vi "Test Comm.vi"() -> ()   [LabVIEW 2021]
uses:
  ChannelCommon/typedef/FIFO Config.ctl
  ChannelCommon/ChannelCommon.lvlib
  CIFChannels/Typedef/Direction.ctl
  CIFChannels/CIFChannels.lvclass
  CIF_NIChn_DAQ_Base.lvclass
  ChannelCommon/typedef/TimeStamps.ctl
  ChannelCommon/typedef/Datatype Waveform.ctl
  ChannelCommon/typedef/New FIFO Instance Response.ctl
panel:
  out "status":string
  out "pass":bool
  out "error out":errorcluster
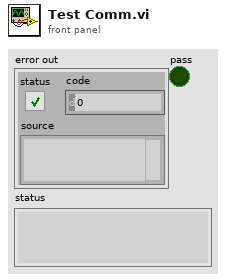
[diagram p1: front panel]
types:
  T1 = typedef "CIFChannels.lvclass/Direction.ctl" = enum16{"Publisher", "Subscriber"}
  T2 = typedef "ChannelCommon.lvlib/New FIFO Instance Response.ctl" = cluster{"Publisher":string, "Custom Data":u8[]}
  T3 = typedef "ChannelCommon.lvlib/TimeStamps.ctl" = cluster{"ClockID":u8, "T0":i64, "T_Out":i64}
  T4 = typedef "ChannelCommon.lvlib/FIFO Config.ctl" = cluster{"Max Bytes/Msg":u64, "Max Msg/FIFO":u64, "Flags":u64}
  T5 = typedef "ChannelCommon.lvlib/Datatype Waveform.ctl" = cluster{"Measurement":dbl[], "dT":dbl, "Timestamp":i64}
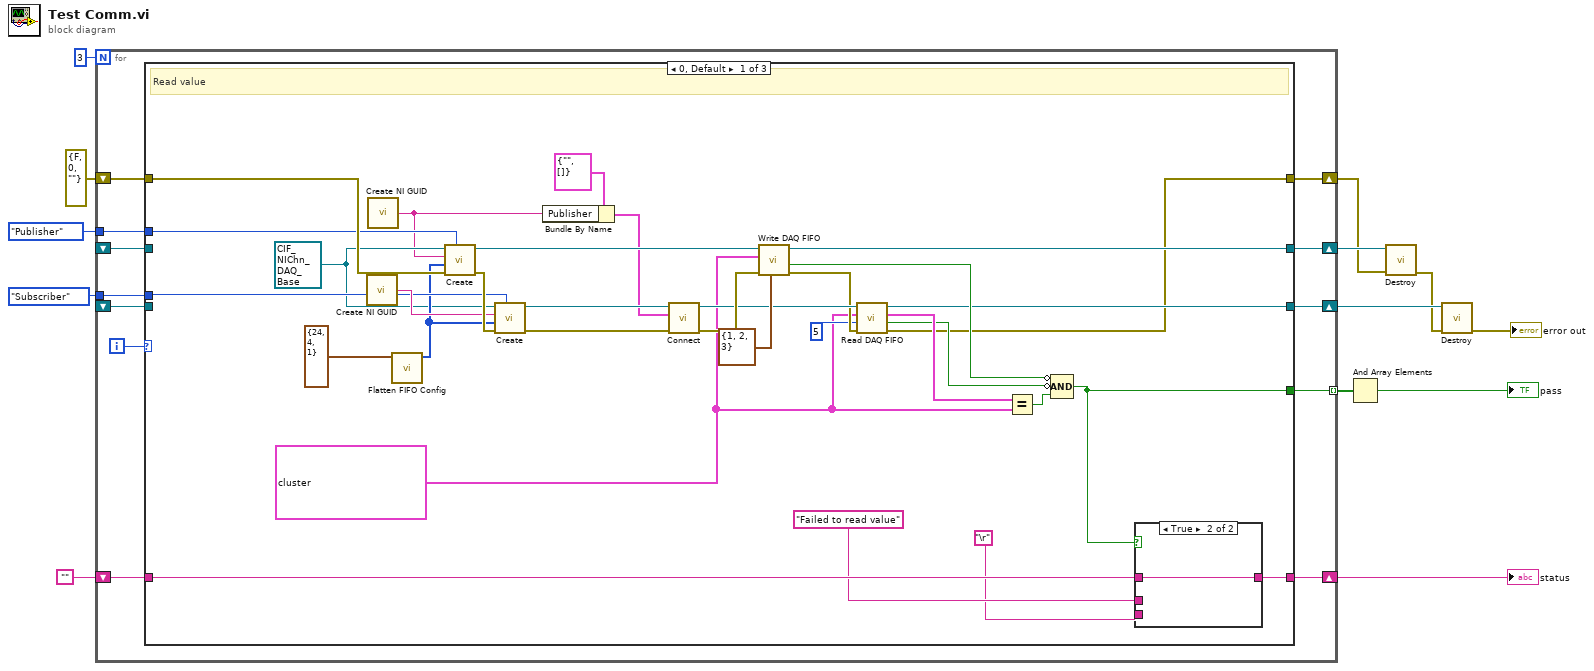
[diagram p0: block diagram]
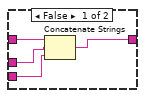
[diagram p2: hidden frame]
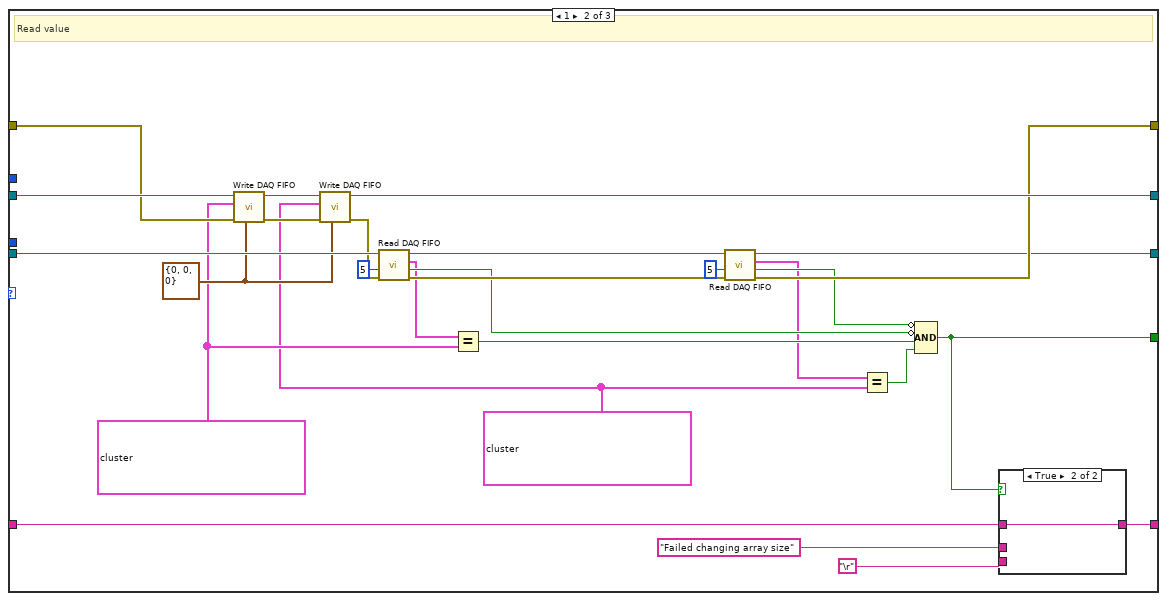
[diagram p3: hidden frame]
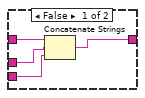
[diagram p4: hidden frame]
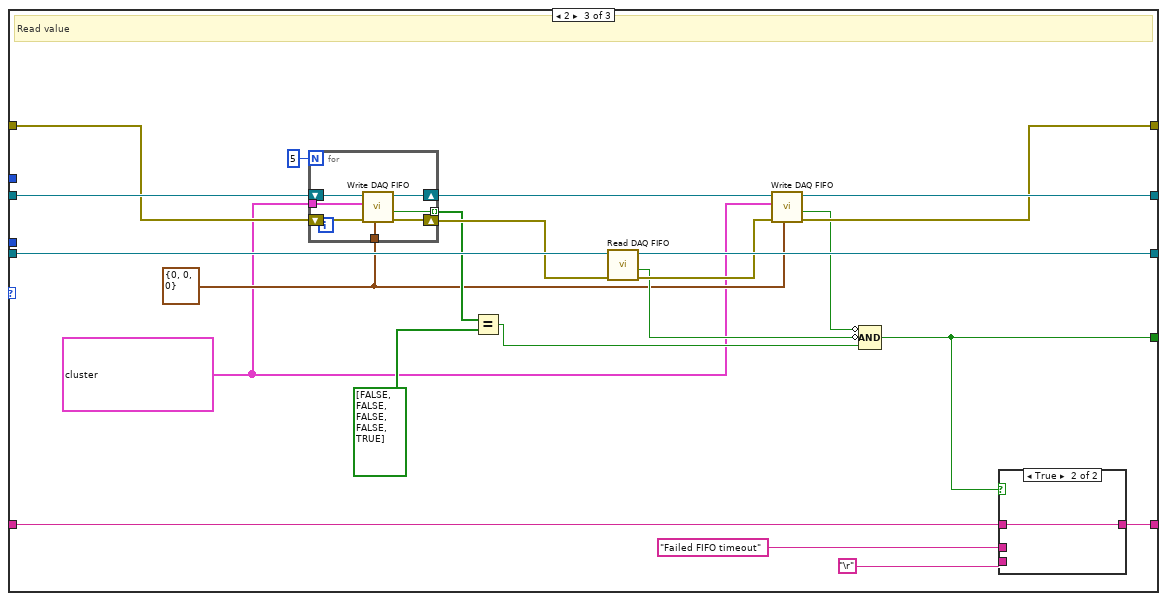
[diagram p5: hidden frame]
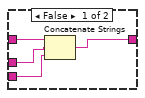
[diagram p6: hidden frame]
diagram:
  n1 = for {
    N: 3 -> [_]
    tunnel: [w25] -> w13 mode=indexing
    shift-right: [w14] -> w3
    shift-left: errorcluster {"status"=FALSE, "code"=0, "source"=""} ("error out") -> [w24]
    shift-right: [w21] -> w9
    shift-left: "" -> [w22]
    tunnel: Direction."Subscriber" ("Direction") -> [w20]
    tunnel: Direction."Publisher" ("Direction") -> [w19]
    shift-right: [w18] -> w5
    shift-left: _ -> [w16]
    shift-right: [w17] -> w4
    shift-left: _ -> [w15]
    i -> [w23]
    n2 = case shown="0, Default" w23 {
      tunnel: [w52 w85 w97] -> w25
      tunnel: w24 -> [w50 w81 w111]
      tunnel: [w30 w74 w103] -> w14
      tunnel: w22 -> [w57 w89 w116]
      tunnel: [w56 w88 w115] -> w21
      tunnel: w20 -> [w48 _ _]
      tunnel: w19 -> [w47 _ _]
      tunnel: [w32 w71 w108] -> w18
      tunnel: [w38 w78 w106] -> w17
      tunnel: w15 -> [_ w82 w112]
      tunnel: w16 -> [_ w77 w109]
      frame 0, Default {
        w42 = refnum<class "CIF_NIChn_DAQ_Base.lvclass"> refnum ("CIF_NIChn_FIFO_DAQ.lvclass")
        w29 = T5[] [{"Measurement"=array[986 elements], "dT"=43.0, "Timestamp"=2}, {"Measurement"=array[1001 elements], "dT"=34.0, "Timestamp"=1}] ("DAQ In")
        # "Read value"
        n3 = call <vilib>:"Create NI GUID.vi"() -> ("NI GUID"=w49:string)
        n4 = call <vilib>:"Create NI GUID.vi"() -> ("NI GUID"=w27:string)
        n5 = call "Flatten FIFO Config.vi"("FIFO Config in"=T4 {"Max Bytes/Msg"=24, "Max Msg/FIFO"=4, "Flags"=1}) -> ("Flattened FIFO Config"=w43:u8[])  [unwired: 10 in]
        n6 = call-dynamic "Create.vi"("Direction"=w47, "error in (no error)"=w50, "Custom Config Data"=w43, "Name"=w27, "CIF_NIChn_FIFO_DAQ in"=w42) -> ("error out"=w51:errorcluster, "CIF_NIChn_FIFO_DAQ out"=w41:refnum<class "CIF_NIChn_DAQ_Base.lvclass">)  [unwired: 5 in]
        n7 = call-dynamic "Create.vi"("Direction"=w48, "error in (no error)"=w51, "Custom Config Data"=w43, "Name"=w49, "CIF_NIChn_FIFO_DAQ in"=w42) -> ("error out"=w45:errorcluster, "CIF_NIChn_FIFO_DAQ out"=w44:refnum<class "CIF_NIChn_DAQ_Base.lvclass">)  [unwired: 5 in]
        n8 = Bundle By Name(cluster=T2 {"Publisher"="", "Custom Data"=[]} ("Connection"), "Publisher"=w27) -> (w26:T2)
        n9 = call-dynamic "Connect.vi"("error in (no error)"=w45, "Connection"=w26, "CIFTag in"=w44) -> ("error out"=w40:errorcluster, "CIFTag out"=w36:refnum<class "CIF_NIChn_DAQ_Base.lvclass">)  [unwired: 7 in]
        n10 = call-dynamic "Write DAQ FIFO.vi"("FIFO Timestamps"=T3 {"ClockID"=1, "T0"=2, "T_Out"=3}, "error in (no error)"=w40, "Data In"=w29, "CIF_NIChn_FIFO_DAQ in"=w41) -> ("error out"=w35:errorcluster, "timed out?"=w37:bool, "CIF_NIChn_FIFO_DAQ out"=w38:refnum<class "CIF_NIChn_DAQ_Base.lvclass">)  [unwired: 4 in, 1 out]
        n11 = call-dynamic "Read DAQ FIFO.vi"("error in (no error)"=w35, "Timeout (ms)"=5, "Data In"=w29, "CIF_NIChn_FIFO_DAQ in"=w36) -> ("error out"=w30:errorcluster, "timed out?"=w31:bool, "Data Out"=w33:T5[], "CIF_NIChn_FIFO_DAQ out"=w32:refnum<class "CIF_NIChn_DAQ_Base.lvclass">)  [unwired: 3 in, 1 out]
        n12 = Equal?(x=w33, y=w29) -> (x = y?=w53:bool)
        n13 = Compound Arithmetic op=AND(invert w37, invert w31, w53) -> (w52:bool)
        n14 = case shown="True" w52 {
          tunnel: w57 -> [w61 w62]
          tunnel: [w58 w62] -> w56
          tunnel: "Failed to read value" -> [w60 _]
          tunnel: "\r" -> [w59 _]
          frame False {
            n15 = Concatenate Strings(w61, w60, w59) -> (w58:string)
          }
          frame True {
          }
        }
      }
      frame 1 {
        w63 = T5[] [{"Measurement"=array[986 elements], "dT"=213.0, "Timestamp"=2}, {"Measurement"=array[1001 elements], "dT"=32.0, "Timestamp"=1}, {"Measurement"=array[988 elements], "dT"=123.0, "Timestamp"=4}] ("DAQ In")
        w64 = T5[] [{"Measurement"=array[986 elements], "dT"=1.0, "Timestamp"=2}, {"Measurement"=array[1001 elements], "dT"=83.0, "Timestamp"=1}, {"Measurement"=array[988 elements], "dT"=78.0, "Timestamp"=4}] ("DAQ In")
        w65 = T3 {"ClockID"=0, "T0"=0, "T_Out"=0} ("FIFO Timestamps")
        # "Read value"
        n16 = call-dynamic "Write DAQ FIFO.vi"("FIFO Timestamps"=w65, "error in (no error)"=w81, "Data In"=w64, "CIF_NIChn_FIFO_DAQ in"=w82) -> ("error out"=w79:errorcluster, "CIF_NIChn_FIFO_DAQ out"=w80:refnum<class "CIF_NIChn_DAQ_Base.lvclass">)  [unwired: 4 in, 2 out]
        n17 = call-dynamic "Write DAQ FIFO.vi"("FIFO Timestamps"=w65, "error in (no error)"=w79, "Data In"=w63, "CIF_NIChn_FIFO_DAQ in"=w80) -> ("error out"=w75:errorcluster, "CIF_NIChn_FIFO_DAQ out"=w78:refnum<class "CIF_NIChn_DAQ_Base.lvclass">)  [unwired: 4 in, 2 out]
        n18 = call-dynamic "Read DAQ FIFO.vi"("error in (no error)"=w75, "Timeout (ms)"=5, "CIF_NIChn_FIFO_DAQ in"=w77) -> ("error out"=w73:errorcluster, "timed out?"=w69:bool, "Data Out"=w66:T5[], "CIF_NIChn_FIFO_DAQ out"=w70:refnum<class "CIF_NIChn_DAQ_Base.lvclass">)  [unwired: 4 in, 1 out]
        n19 = Equal?(x=w66, y=w64) -> (x = y?=w83:bool)
        n20 = call-dynamic "Read DAQ FIFO.vi"("error in (no error)"=w73, "Timeout (ms)"=5, "CIF_NIChn_FIFO_DAQ in"=w70) -> ("error out"=w74:errorcluster, "timed out?"=w68:bool, "Data Out"=w67:T5[], "CIF_NIChn_FIFO_DAQ out"=w71:refnum<class "CIF_NIChn_DAQ_Base.lvclass">)  [unwired: 4 in, 1 out]
        n21 = Equal?(x=w67, y=w63) -> (x = y?=w84:bool)
        n22 = Compound Arithmetic op=AND(invert w68, invert w69, w83, w84) -> (w85:bool)
        n23 = case shown="True" w85 {
          tunnel: w89 -> [w93 w94]
          tunnel: [w90 w94] -> w88
          tunnel: "Failed changing array size" -> [w92 _]
          tunnel: "\r" -> [w91 _]
          frame False {
            n24 = Concatenate Strings(w93, w92, w91) -> (w90:string)
          }
          frame True {
          }
        }
      }
      frame 2 {
        w95 = T5[] [{"Measurement"=array[986 elements], "dT"=43.0, "Timestamp"=2}, {"Measurement"=array[1001 elements], "dT"=34.0, "Timestamp"=1}] ("DAQ In")
        w96 = T3 {"ClockID"=0, "T0"=0, "T_Out"=0} ("FIFO Timestamps")
        # "Read value"
        n25 = for {
          N: 5 -> [_]
          tunnel: w95 -> [w121]
          tunnel: w96 -> [w120]
          shift-right: [w119] -> w107
          shift-left: w112 -> [w123]
          tunnel: [w118] -> w102 mode=indexing
          shift-right: [w117] -> w105
          shift-left: w111 -> [w122]
          n26 = call-dynamic "Write DAQ FIFO.vi"("FIFO Timestamps"=w120, "error in (no error)"=w122, "Data In"=w121, "CIF_NIChn_FIFO_DAQ in"=w123) -> ("error out"=w117:errorcluster, "timed out?"=w118:bool, "CIF_NIChn_FIFO_DAQ out"=w119:refnum<class "CIF_NIChn_DAQ_Base.lvclass">)  [unwired: 4 in, 1 out]
        }
        n27 = Equal?(x=w102, y=bool[] [FALSE, FALSE, FALSE, FALSE, TRUE]) -> (x = y?=w98:bool)
        n28 = call-dynamic "Read DAQ FIFO.vi"("error in (no error)"=w105, "CIF_NIChn_FIFO_DAQ in"=w109) -> ("error out"=w104:errorcluster, "timed out?"=w100:bool, "CIF_NIChn_FIFO_DAQ out"=w108:refnum<class "CIF_NIChn_DAQ_Base.lvclass">)  [unwired: 5 in, 2 out]
        n29 = call-dynamic "Write DAQ FIFO.vi"("FIFO Timestamps"=w96, "error in (no error)"=w104, "Data In"=w95, "CIF_NIChn_FIFO_DAQ in"=w107) -> ("error out"=w103:errorcluster, "timed out?"=w99:bool, "CIF_NIChn_FIFO_DAQ out"=w106:refnum<class "CIF_NIChn_DAQ_Base.lvclass">)  [unwired: 4 in, 1 out]
        n30 = Compound Arithmetic op=AND(invert w99, invert w100, w98) -> (w97:bool)
        n31 = case shown="True" w97 {
          tunnel: w116 -> [w127 w128]
          tunnel: [w124 w128] -> w115
          tunnel: "Failed FIFO timeout" -> [w126 _]
          tunnel: "\r" -> [w125 _]
          frame False {
            n32 = Concatenate Strings(w127, w126, w125) -> (w124:string)
          }
          frame True {
          }
        }
      }
    }
  }
  "status" <- w9
  n33 = And Array Elements(Boolean array=w13) -> (logical AND=→"pass":bool)
  n34 = call-dynamic "Destroy.vi"("error in (no error)"=w3, "CIF_NIChn_FIFO_DAQ in"=w4) -> ("error out"=w2:errorcluster)  [unwired: 8 in, 1 out]
  n35 = call-dynamic "Destroy.vi"("error in (no error)"=w2, "CIF_NIChn_FIFO_DAQ in"=w5) -> ("error out"=→"error out":errorcluster)  [unwired: 8 in, 1 out]
